vi "Get Term Type.vi"(9 "Term Types":cluster{"Type":variant, "Id":string}[](array[cluster]), 10 "ID":string) -> (2 "Type":variant)   [LabVIEW 2015, in "Scripting.lvlib"]
uses:
  Scripting.lvlib
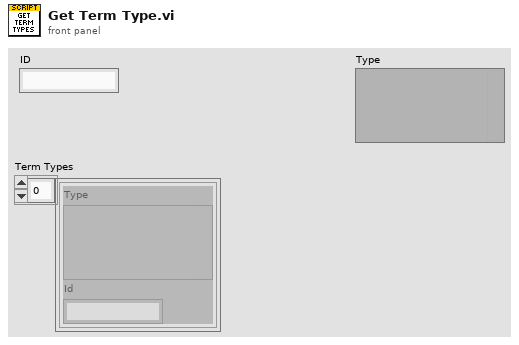
[diagram p1: front panel]
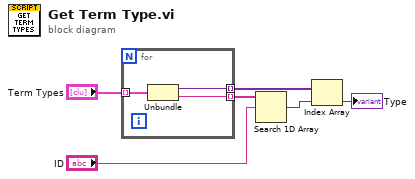
[diagram p0: block diagram]
diagram:
  n1 = for {
    tunnel: "Term Types" -> [w9] mode=indexing
    tunnel: [w8] -> w2 mode=indexing
    tunnel: [w7] -> w5 mode=indexing
    n2 = Unbundle(w9) -> ("Type"=w8:variant, "Id"=w7:string)
  }
  n3 = Search 1D Array(1D array=w5, element="ID") -> (index of element=w3:i32)  [unwired: 1 in]
  n4 = Index Array(array=w2, index=w3) -> (element=→"Type":variant)
